vi "Capture Sorted Peak Index (Angle) (SubVI).vi"(8 "Angle":fxp<+/-,16,3> format="%.14g", 9 "Peak Index":u16, 10 "Dip Valid?":bool, 11 "Peak Count":u16) -> (0 "Angle Array":fxp<+/-,16,3>[](array[numeric]) format="%.14g", 3 "Sorted Peak Index":u16[](array[numeric]))   [LabVIEW 2015]
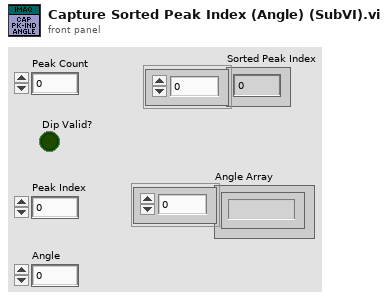
[diagram p1: front panel]
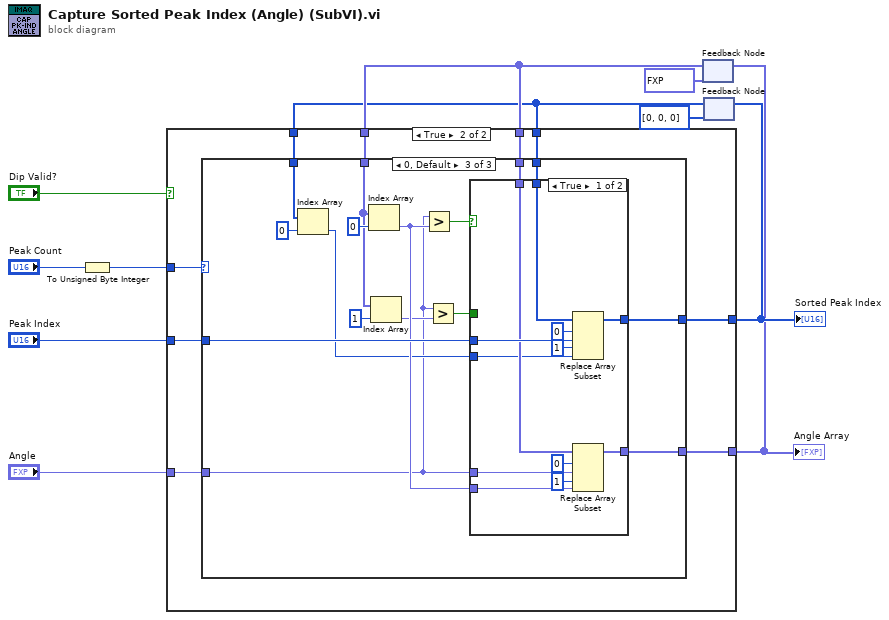
[diagram p0: block diagram]
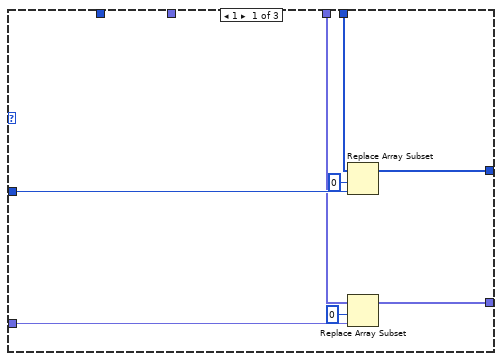
[diagram p3: hidden frame]
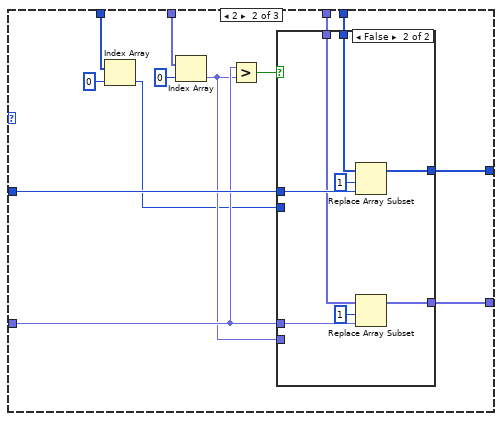
[diagram p4: hidden frame]
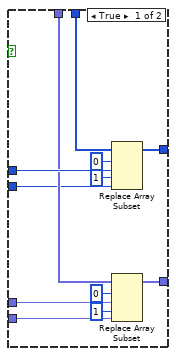
[diagram p5: hidden frame]
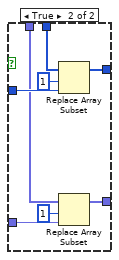
[diagram p7: hidden frame]
diagram:
  n1 = To Unsigned Byte Integer(number="Peak Count") -> (unsigned 8bit integer=w1:u8)
  n2 = feedback #1(fxp<+/-,16,3>[] [0.0, 0.0, 0.0]) -> (w3:fxp<+/-,16,3>[])
  n3 = feedback #2(u16[] [0, 0, 0]) -> (w2:u16[])
  n4 = case shown="True" "Dip Valid?" {
    tunnel: "Peak Index" -> [_ w22]
    tunnel: "Angle" -> [_ w19]
    tunnel: [w13 w21] -> w6
    tunnel: [w12 w20] -> w4
    tunnel: w1 -> [_ w16]
    tunnel: w2 -> [w13 w18]
    tunnel: w3 -> [w12 w17]
    tunnel: w3 -> [_ w15]
    tunnel: w2 -> [_ w14]
    frame False {
    }
    frame True {
      n5 = case shown="0, Default" w16 {
        tunnel: w22 -> [w30 w43 w79]
        tunnel: [w29 w42 w78] -> w21
        tunnel: [w28 w41 w77] -> w20
        tunnel: w19 -> [w27 w36 w64]
        tunnel: w18 -> [w26 w40 w76]
        tunnel: w17 -> [w25 w39 w75]
        tunnel: w15 -> [_ w38 w65]
        tunnel: w14 -> [_ w34 w72]
        frame 1 {
          n6 = Replace Array Subset(array=w26, new element=w30, index=0) -> (w29:u16[])
          n7 = Replace Array Subset(array=w25, new element=w27, index=0) -> (w28:fxp<+/-,16,3>[])
        }
        frame 2 {
          n8 = Index Array(array=w34, index=0) -> (element=w31:u16)
          n9 = Index Array(array=w38, index=0) -> (element=w32:fxp<+/-,16,3>)
          n10 = Greater?(x=w36, y=w32) -> (0:w35:bool)
          n11 = case shown="False" w35 {
            tunnel: w43 -> [w55 w63]
            tunnel: [w54 w62] -> w42
            tunnel: [w53 w61] -> w41
            tunnel: w40 -> [w52 w60]
            tunnel: w39 -> [w51 w59]
            tunnel: w36 -> [w49 w57]
            tunnel: w32 -> [w46 _]
            tunnel: w31 -> [w44 _]
            frame True {
              n12 = Replace Array Subset(array=w52, new element #1=w55, index #1=0 ("index"), new element #2=w44, index #2=1 ("index")) -> (w54:u16[])
              n13 = Replace Array Subset(array=w51, new element #1=w49, index #1=0 ("index"), new element #2=w46, index #2=1 ("index")) -> (w53:fxp<+/-,16,3>[])
            }
            frame False {
              n14 = Replace Array Subset(array=w60, new element=w63, index=1) -> (w62:u16[])
              n15 = Replace Array Subset(array=w59, new element=w57, index=1) -> (w61:fxp<+/-,16,3>[])
            }
          }
        }
        frame 0, Default {
          n16 = Index Array(array=w72, index=0) -> (element=w69:u16)
          n17 = Index Array(array=w65, index=0) -> (element=w70:fxp<+/-,16,3>)
          n18 = Index Array(array=w65, index=1) -> (element=w68:fxp<+/-,16,3>)
          n19 = Greater?(x=w64, y=w70) -> (0:w73:bool)
          n20 = Greater?(x=w64, y=w68) -> (0:w66:bool)
          n21 = case shown="True" w73 {
            tunnel: w79 -> [w91 w98]
            tunnel: [w90 w97] -> w78
            tunnel: [w89 w96] -> w77
            tunnel: w76 -> [w88 w95]
            tunnel: w75 -> [w87 w94]
            tunnel: w64 -> [w85 w93]
            tunnel: w70 -> [w82 _]
            tunnel: w69 -> [w80 _]
            tunnel: w66 -> [_ w92]
            frame True {
              n22 = Replace Array Subset(array=w88, new element #1=w91, index #1=0 ("index"), new element #2=w80, index #2=1 ("index")) -> (w90:u16[])
              n23 = Replace Array Subset(array=w87, new element #1=w85, index #1=0 ("index"), new element #2=w82, index #2=1 ("index")) -> (w89:fxp<+/-,16,3>[])
            }
            frame False {
              n24 = case shown="False" w92 {
                tunnel: w98 -> [_ w108]
                tunnel: [w100 w107] -> w97
                tunnel: [w99 w106] -> w96
                tunnel: w95 -> [w100 w105]
                tunnel: w94 -> [w99 w104]
                tunnel: w93 -> [_ w102]
                frame False {
                }
                frame True {
                  n25 = Replace Array Subset(array=w105, new element=w108, index=1) -> (w107:u16[])
                  n26 = Replace Array Subset(array=w104, new element=w102, index=1) -> (w106:fxp<+/-,16,3>[])
                }
              }
            }
          }
        }
      }
    }
  }
  "Sorted Peak Index" <- w6
  "Angle Array" <- w4
  n27 = feedback-in #1(w4) -> ()
  n28 = feedback-in #2(w6) -> ()
